vi "Set Engine Rate.vi"(8 "error in (no error)":errorcluster, 10 "Engine Rate (Hz)":dbl, 11 "Node Ptr in":T1 format="%.0x") -> (0 "error out":errorcluster, 3 "Node Ptr out":T1=18446744073709551615 format="%.0x")   [LabVIEW 2019, in "TimingDRV System Explorer.lvlib"]
uses:
  TimingDRV System Explorer.lvlib
  <vilib>/NI VeriStand/Custom Device API/Custom Device Item Ref.ctl
  NationalInstruments.VeriStand.SystemDefinitionAPI
  NationalInstruments.VeriStand.SystemStorage
  <vilib>/NI VeriStand/Custom Device API/Custom Device API.lvlib
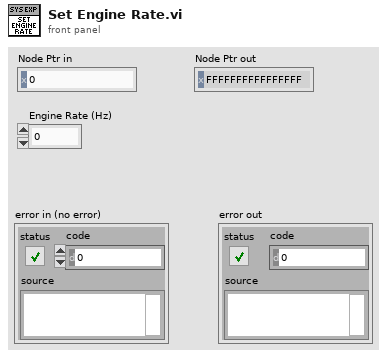
[diagram p1: front panel]
types:
  T1 = typedef "Custom Device API.lvlib/Custom Device Item Ref.ctl" = u64
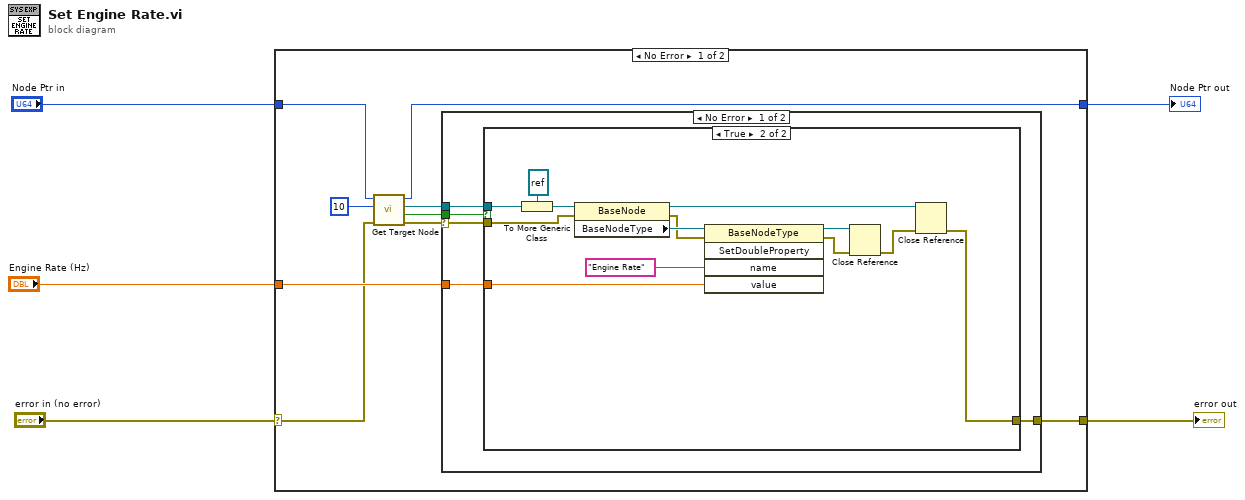
[diagram p0: block diagram]
diagram:
  n1 = case shown="No Error" "error in (no error)" {
    selector: "error in (no error)" -> [w8 w36]
    tunnel: "Engine Rate (Hz)" -> [w14 _]
    tunnel: "Node Ptr in" -> [w10 w35]
    tunnel: [w7 w36] -> w2
    tunnel: [w6 w35] -> w1
    frame No Error {
      n2 = call "Get Target Node.vi"("error in (no error)"=w8, "Max search depth"=10, "Node Ptr in"=w10) -> ("error out"=w9:errorcluster, "Found?"=w12:bool, "Target Ref out"=w13:refnum<k24>, "Node Ptr out"=w6:T1)  [unwired: 5 in]
      n3 = case shown="No Error" w9 {
        selector: w9 -> [w16 w34]
        tunnel: w14 -> [w19 _]
        tunnel: w13 -> [w18 _]
        tunnel: w12 -> [w17 _]
        tunnel: [w15 w34] -> w7
        frame No Error {
          n4 = case shown="True" w17 {
            tunnel: w18 -> [_ w33]
            tunnel: w19 -> [_ w28]
            tunnel: w16 -> [w20 w22]
            tunnel: [w20 w21] -> w15
            frame False {
            }
            frame True {
              n5 = To More Generic Class(target class=refnum<k24> refnum ("reference out"), reference=w33) -> (generic class reference=w31:refnum<k24>)
              n6 = property class="BaseNode"(reference=w31, error in=w22) -> (reference out=w27:refnum<k24>, error out=w24:errorcluster, "BaseNodeType"=w30:refnum<k24>)
              n7 = invoke class="BaseNodeType" method="SetDoubleProperty"(reference=w30, error in=w24, "name"="Engine Rate", "value"=w28) -> (reference out=w25:refnum<k24>, error out=w26:errorcluster)  [unwired: 1 in, 3 out]
              n8 = Close Reference(reference=w25, error in (no error)=w26) -> (error out=w23:errorcluster)
              n9 = Close Reference(reference=w27, error in (no error)=w23) -> (error out=w21:errorcluster)
            }
          }
        }
        frame Error {
        }
      }
    }
    frame Error {
    }
  }
  "error out" <- w2
  "Node Ptr out" <- w1
